vi "Read Club ID.vi"(8 "error in (no error)":errorcluster, 11 "Strava curl in":refnum<class "Strava curl.lvclass">) -> (0 "error out":errorcluster, 2 "Club ID":string, 3 "Strava curl out":refnum<class "Strava curl.lvclass">)   [LabVIEW 2020, in "Strava curl.lvclass"]
uses:
  Strava curl.lvclass
  Strava curl.lvclass/Strava curl.ctl
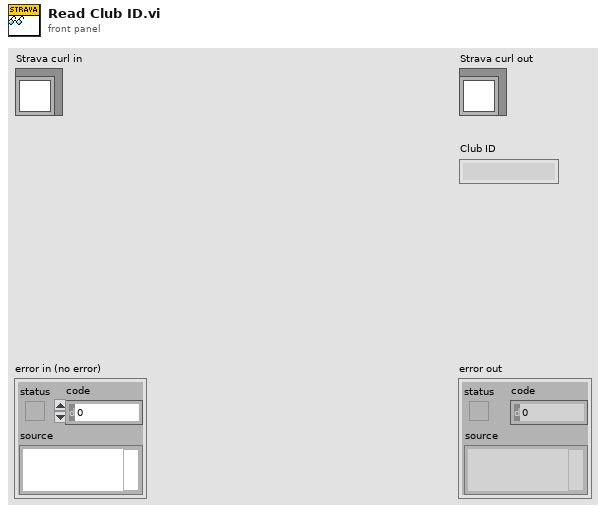
[diagram p1: front panel]
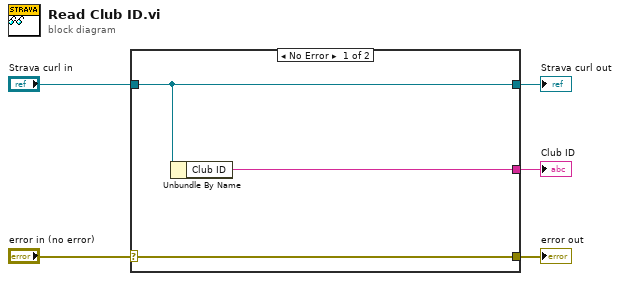
[diagram p0: block diagram]
diagram:
  n1 = case shown="No Error" "error in (no error)" {
    selector: "error in (no error)" -> [w8 w9]
    tunnel: [w8 w9] -> w4
    tunnel: [w7 w10] -> w2
    tunnel: "Strava curl in" -> [w7 w10]
    tunnel: [w6 _] -> w1
    frame No Error {
      n2 = Unbundle By Name(w7) -> ("Club ID"=w6:string)
    }
    frame Error {
    }
  }
  "error out" <- w4
  "Strava curl out" <- w2
  "Club ID" <- w1
